vi "build Application.vi"() -> ()   [LabVIEW 2014]
uses:
  <vilib>/AppBuilder/AB_API_Simple/Build (path).vi
  <vilib>/AppBuilder/AB_API_Simple/NI_App_Builder_API.lvlib
panel:
  out "error out":errorcluster
  out "Generated files":path[](array[path])
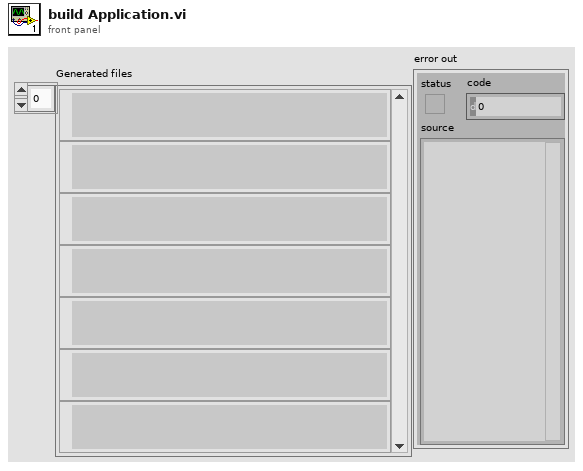
[diagram p1: front panel]
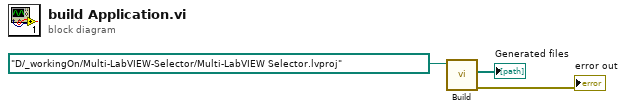
[diagram p0: block diagram]
diagram:
  n1 = call-poly <vilib>:"Build.vi"("Path to project"=path "D:/_workingOn/Multi-LabVIEW-Selector/Multi-LabVIEW Selector.lvproj") -> ("error out"=→"error out":errorcluster, "Generated files"=→"Generated files":path[])  [unwired: 9 in]
